vi "获取频响函数.vi"() -> ()   [LabVIEW 2014]
uses:
  <vilib>/Analysis/4window.llb/windowTd.ctl
  <vilib>/DAQmx/read.llb/DAQmx Read (Analog 1D Wfm NChan NSamp).vi
  <vilib>/DAQmx/create/channels.llb/DAQmx Create Channel (AI-Voltage-Basic).vi
  <vilib>/DAQmx/configure/timing.llb/DAQmx Timing (Sample Clock).vi
  <vilib>/DAQmx/miscellaneous.llb/DAQmx Fill In Error Info.vi
  <resource>/objmgr/daqmx.rc
  <vilib>/Analysis/NI_AALPro.lvlib
panel:
  out "响应信号":waveform(dbl)(graph)
  out "激振信号":waveform(dbl)(graph)
  in  "设置平均计数":i32
  out "当前平均计数":i32
  in  "dB On (F)":bool
  in  "averaging mode":T1(ring)
  in  "number of averages":u32
  in  "view":T2 caption="查看"
  in  "window":T3=1 caption="窗" items=["矩形"=0, "Hanning"=1, "Hamming"=2, "Blackman-Harris"=3, "Exact Blackman"=4, "Blackman"=5, "Flat Top"=6, "4阶Blackman-Harris "=7, "7阶Blackman-Harris"=8, "Low Sidelobe"=9, "Blackman Nuttall"=11, "三角"=30, "Bartlett-Hanning"=31, "Bohman"=32, "Parzen"=33, "Welch"=34, "Kaiser"=60, "Dolph-Chebyshev"=61, "高斯"=62]
  in  "删除上一波形":bool caption="删除上一次波形"
  in  "FRF Mode":enum16{"H1", "H2", "H3"}(ring) caption="FRF模式"
  in  "预触发":i32
  in  "阈值":dbl format="%#_13g"
  in  "获得激振通道":i32
  in  "采样数":i32
  in  "units 2":i32(ring)=10348 caption="单位" items=["伏特"=10348, "来自自定义换算"=10065]
  in  "units":i32(ring)=10348 caption="单位" items=["伏特"=10348, "来自自定义换算"=10065]
  in  "sample mode 2":i32(ring)=10178 caption="采样模式" items=["有限采样"=10178, "连续采样"=10123, "硬件定时单点"=12522]
  in  "rate 2":dbl=1000.0 caption="速率" format="%0.2f"
  in  "input terminal configuration 3":i32(ring)=-1 caption="输入接线端配置" items=["默认"=-1, "RSE"=10083, "NRSE"=10078, "差分"=10106, "伪差分"=12529]
  in  "DAQmx物理通道 2":tag
  in  "input terminal configuration 2":i32(ring)=-1 caption="输入接线端配置" items=["默认"=-1, "RSE"=10083, "NRSE"=10078, "差分"=10106, "伪差分"=12529]
  in  "DAQmx物理通道":tag
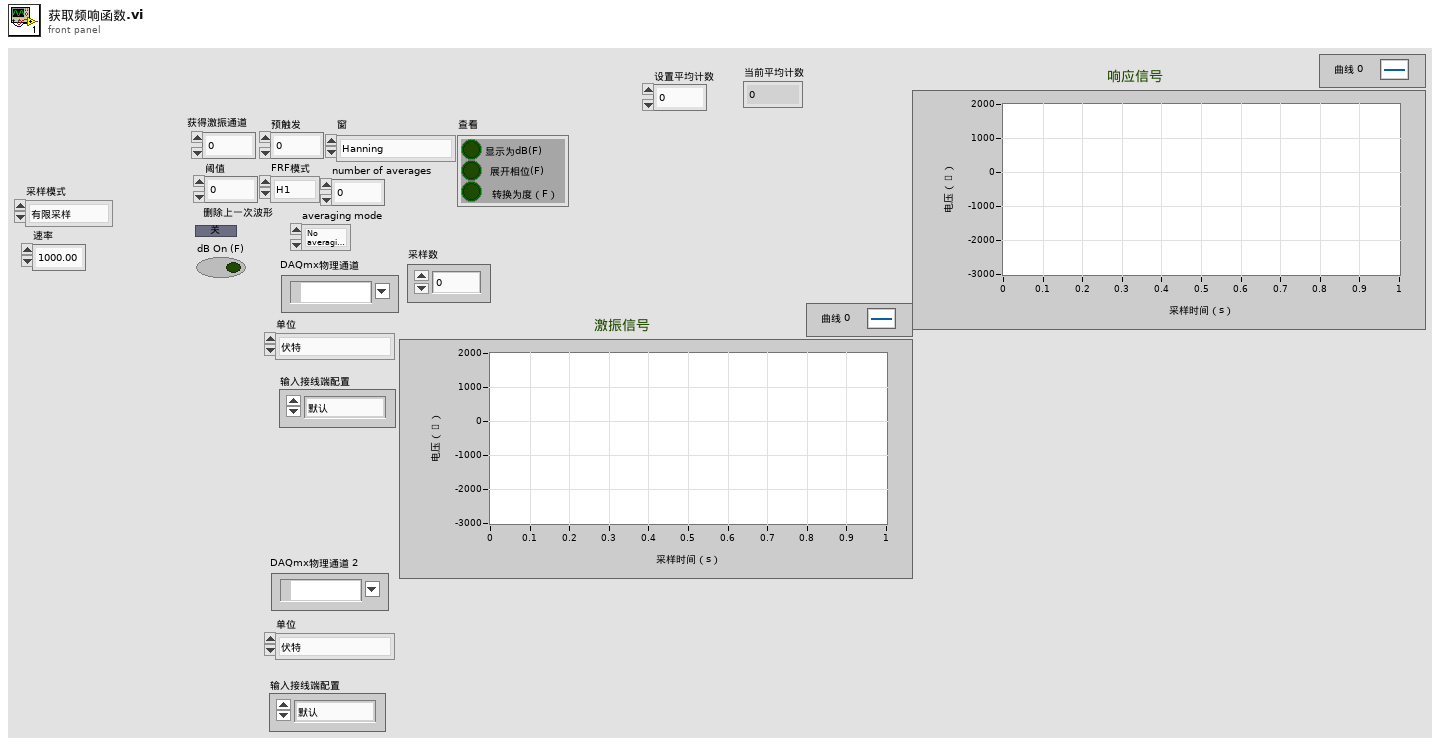
[diagram p1: front panel]
types:
  T1 = enum16{"No averaging", "Vector averaging", "RMS averaging", "Peak hold"}
  T2 = cluster{"dB On (F)":bool, "unwrap phase (F)":bool, "convert to degree (F)":bool}
  T3 = typedef "NI_AALPro.lvlib/windowTd.ctl" = u32
  T4 = cluster{"number of averages":u32, "averaging mode":enum16{"No averaging", "Vector averaging", "RMS averaging", "Peak hold"}, "window":T3, "view":cluster{"dB On (F)":bool, "unwrap phase (F)":bool, "convert to degree (F)":bool}, "设置平均计数":i32}
  T5 = cluster{"averaging mode":enum16{"No averaging", "Vector averaging", "RMS averaging", "Peak hold"}, "weighting mode":enum16{"Linear", "Exponential"}, "number of averages":u32}
  T6 = cluster{"magnitude":cluster{"f0":dbl, "df":dbl, "magnitude":dbl[]}, "phase":cluster{"f0":dbl, "df":dbl, "phase":dbl[]}, "coherence":cluster{"f0":dbl, "df":dbl, "coherence":dbl[]}}
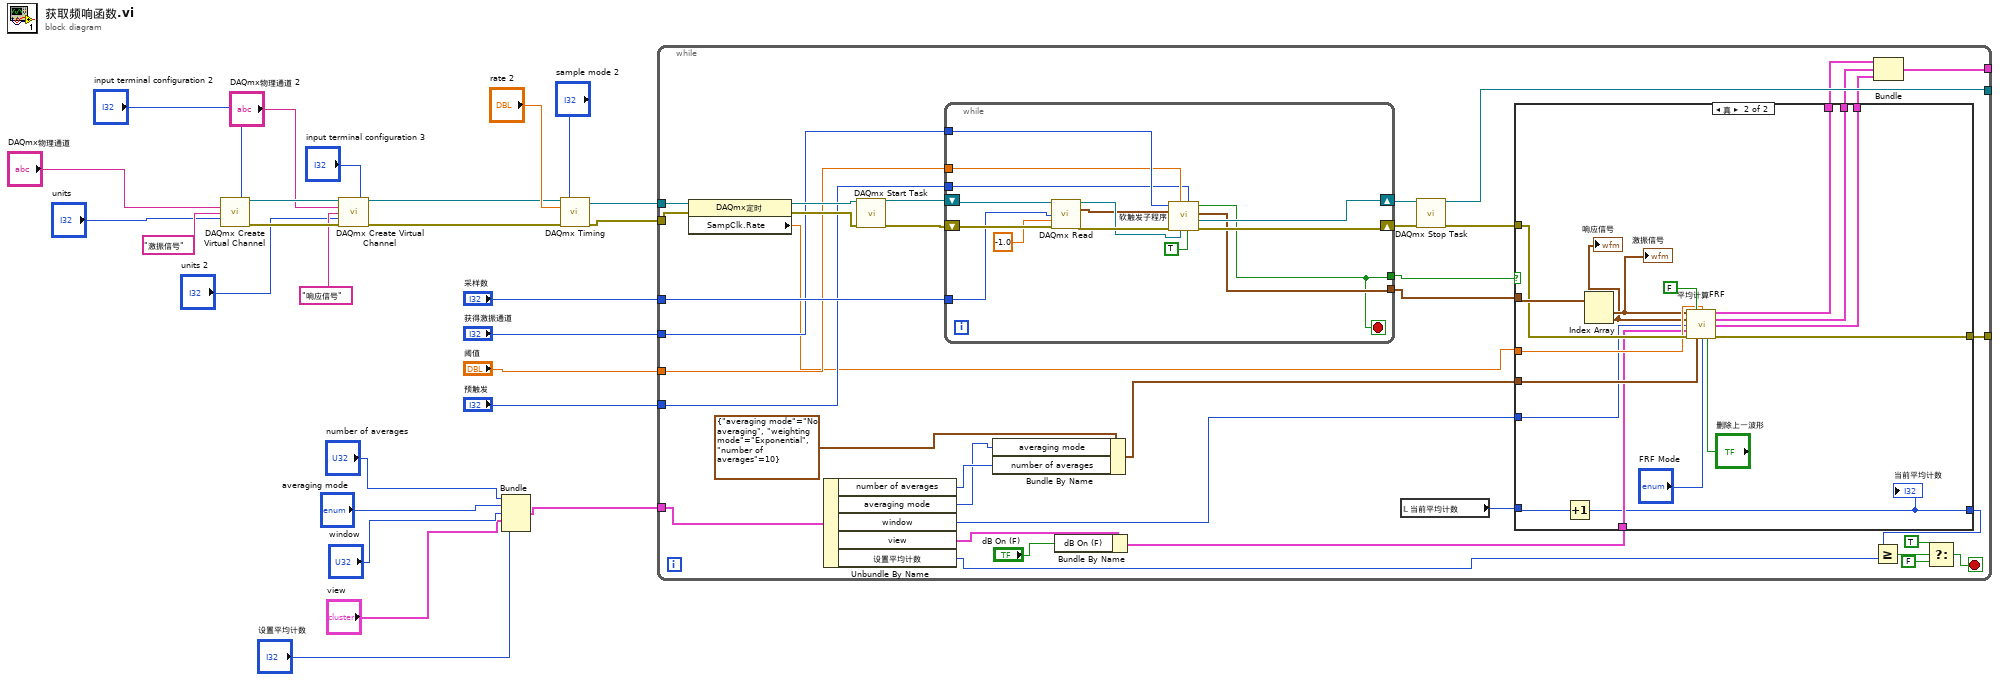
[diagram p0: block diagram]
diagram:
  n1 = call-poly <vilib>:"DAQmx Create Virtual Channel.vi"("input terminal configuration"="input terminal configuration 2", "physical channels"="DAQmx物理通道", "name to assign"="激振信号", "units"="units") -> ("task out"=w23:refnum<k21>, "error out"=w22:errorcluster)  [unwired: 10 in]
  n2 = call-poly <vilib>:"DAQmx Create Virtual Channel.vi"("task in"=w23, "input terminal configuration"="input terminal configuration 3", "physical channels"="DAQmx物理通道 2", "name to assign"="响应信号", "units"="units 2", "error in"=w22) -> ("task out"=w16:refnum<k21>, "error out"=w15:errorcluster)  [unwired: 8 in]
  n3 = Bundle("number of averages"="number of averages", "averaging mode"="averaging mode", "window"="window", "view"="view", "设置平均计数"="设置平均计数") -> (w3:T4)  [unwired: 1 in]
  n4 = call-poly <vilib>:"DAQmx Timing.vi"("task/channels in"=w16, "sample mode"="sample mode 2", "rate"="rate 2", "error in"=w15) -> ("task out"=w12:refnum<k21>, "error out"=w11:errorcluster)  [unwired: 10 in]
  n5 = while {
    tunnel: w12 -> [w64]
    tunnel: w11 -> [w63]
    tunnel: "采样数" -> [w58]
    tunnel: "获得激振通道" -> [w57]
    tunnel: "阈值" -> [w56]
    tunnel: "预触发" -> [w55]
    tunnel: [w52] -> _
    tunnel: [w45] -> _
    tunnel: w3 -> [w44]
    tunnel: [w27] -> _
    stop <- w31 stop-if-true
    n6 = property class="DAQmx定时"(reference=w64, error in=w63) -> (reference out=w62:refnum<k21>, error out=w61:errorcluster, "SampClk.Rate"=w48:dbl)
    n7 = Unbundle By Name(w44) -> ("number of averages"=w43:u32, "averaging mode"=w42:T1, "window"=w41:T3, "view"=w40:T2, "设置平均计数"=w35:i32)
    n8 = call <vilib>:"DAQmx Start Task.vi"("task/channels in"=w62, "error in"=w61) -> ("task out"=w60:refnum<k21>, "error out"=w59:errorcluster)  [unwired: 12 in]
    n9 = while {
      shift-right: [w87] -> w54
      shift-left: w60 -> [w96]
      shift-right: [w93] -> w53
      shift-left: w59 -> [w95]
      tunnel: w58 -> [w90]
      tunnel: [w82] -> w50
      tunnel: [w86] -> w49
      tunnel: w57 -> [w85]
      tunnel: w56 -> [w84]
      tunnel: w55 -> [w83]
      stop <- w82 stop-if-true
      n10 = call-poly <vilib>:"DAQmx Read.vi"("task/channels in"=w96, "number of samples per channel"=w90, "timeout"=-1.0, "error in"=w95) -> ("task out"=w92:refnum<k21>, "data"=w91:waveform(dbl)[], "error out"=w94:errorcluster)  [unwired: 9 in]
      n11 = call "软触发子程序.vi"("触发"=TRUE, "预触发长度"=w83, "task/channels in"=w92, "阈值"=w84, "error in (no error)"=w94, "激振信号"=w91, "激振通道"=w85) -> ("error out"=w93:errorcluster, "task out"=w87:refnum<k21>, "ÏìÓ¦ÐÅº3"=w86:waveform(dbl)[], "模拟触发"=w82:bool)  [unwired: 1 in]
    }
    n12 = Bundle By Name(cluster=T5 {"averaging mode"=enum."No averaging", "weighting mode"=enum."Exponential", "number of averages"=10} ("averaging parameters"), "averaging mode"=w42, "number of averages"=w43) -> (w46:T5)
    n13 = Bundle By Name(cluster=w40, "dB On (F)"="dB On (F)") -> (w38:T2)
    n14 = local read "当前平均计数"() -> (w37:i32)
    n15 = call <vilib>:"DAQmx Stop Task.vi"("task/channels in"=w54, "error in"=w53) -> ("task out"=w52:refnum<k21>, "error out"=w51:errorcluster)  [unwired: 12 in]
    n16 = case shown="真" w50 {
      tunnel: w51 -> [_ w78]
      tunnel: w49 -> [_ w81]
      tunnel: w48 -> [_ w74]
      tunnel: w46 -> [_ w80]
      tunnel: [_ w77] -> w45
      tunnel: w41 -> [_ w73]
      tunnel: w38 -> [_ w72]
      tunnel: w37 -> [_ w71]
      tunnel: [_ w70] -> w36
      tunnel: [_ w69] -> w30
      tunnel: [_ w68] -> w29
      tunnel: [_ w67] -> w28
      frame False {
      }
      frame True {
        n17 = Increment(x=w71) -> (x+1=w70:i32)
        "当前平均计数" <- w70
        n18 = Index Array(array=w81) -> (element #1=w66:waveform(dbl), element #2=w65:waveform(dbl))  [unwired: 2 in]
        "激振信号" <- w66
        "响应信号" <- w65
        n19 = call "平均计算FRF.vi"("time signal X"=w66, "restart averaging (F)"=FALSE, "window parameter"=w74, "time signal Y"=w65, "window"=w73, "view"=w72, "error in (no error)"=w78, "averaging parameters"=w80, "FRF Mode"="FRF Mode", "删除上一波形"="删除上一波形") -> ("magnitude"=w69:cluster{"f0":dbl, "df":dbl, "magnitude":dbl[]}, "phase"=w68:cluster{"f0":dbl, "df":dbl, "phase":dbl[]}, "coherence"=w67:cluster{"f0":dbl, "df":dbl, "coherence":dbl[]}, "error out"=w77:errorcluster)  [unwired: 2 out]
      }
    }
    n20 = Greater Or Equal?(x=w36, y=w35) -> (x >= y?=w34:bool)
    n21 = Bundle("magnitude"=w30, "phase"=w29, "coherence"=w28) -> (w27:T6)  [unwired: 1 in]
    n22 = Select(t=TRUE, s=w34, f=FALSE) -> (s? t:f=w31:bool)
  }
